vi "Write Plugin Connection Map.vi"(8 "error in (no error)":errorcluster, 10 "Plugin Connection Map":T1, 11 "CIF_UI in":refnum<class "CIF_UI.lvclass">) -> (0 "error out":errorcluster, 3 "CIF_UI out":refnum<class "CIF_UI.lvclass">)   [LabVIEW 2021, in "CIF_UI.lvclass"]
uses:
  CIF_UI.lvclass
  Typedef/Plugin Connection Map.ctl
  Typedef/Plugin Connections.ctl
  <vilib>/gRPC/LabVIEW gRPC Library/Shared/grpcId.ctl
  CIFPluginManager/CIFPluginManager/gRPC/CIF_Manager_client/RPC Messages/cif_manager_PluginInfo.ctl
  CIFPluginManager/CIFPluginManager/gRPC/CIF_Manager_client/RPC Messages/cif_manager_PluginVersion.ctl
  CIFPluginManager/CIFPluginManager/gRPC/CIF_Manager_client/RPC Messages/cif_plugincore_StatusData.ctl
  CIFPluginManager/CIFPluginManager/gRPC/CIF_Manager_client/RPC Messages/cif_plugincore_StatusData_State.ctl
  CIFPluginManager/CIFPluginManager/gRPC/CIF_Manager_client/RPC Messages/cif_plugincore_TimingStatistics.ctl
  CIFPluginManager/CIFPluginManager/gRPC/CIF_Manager_client/RPC Messages/cif_plugincore_TimingStatsBasic.ctl
  CIFPluginManager/CIFPluginManager/gRPC/CIF_Manager_client/RPC Messages/cif_plugincore_FifoStatistics.ctl
  CIFPluginManager/CIFPluginManager/gRPC/CIF_Manager_client/RPC Messages/cif_plugincore_Error.ctl
  CIFPluginManager/CIFPluginManager/gRPC/CIF_Manager_client/RPC Messages/cif_plugincore_MonitorDoubles.ctl
  CIFPluginManager/CIFPluginManager/gRPC/CIF_Manager_client/RPC Messages/cif_plugincore_MonitorU64.ctl
  CIFPluginManager/CIFPluginManager/gRPC/CIF_Manager_client/RPC Messages/cif_plugincore_MonitorI64.ctl
  CIF_UI.lvclass/CIF_UI.ctl
  CIFPluginManager/CIFPluginManager/gRPC/CIF_Manager_client/CIF_Manager_client.lvlib
  <vilib>/gRPC/LabVIEW gRPC Library/grpc-lvsupport-release.lvlib
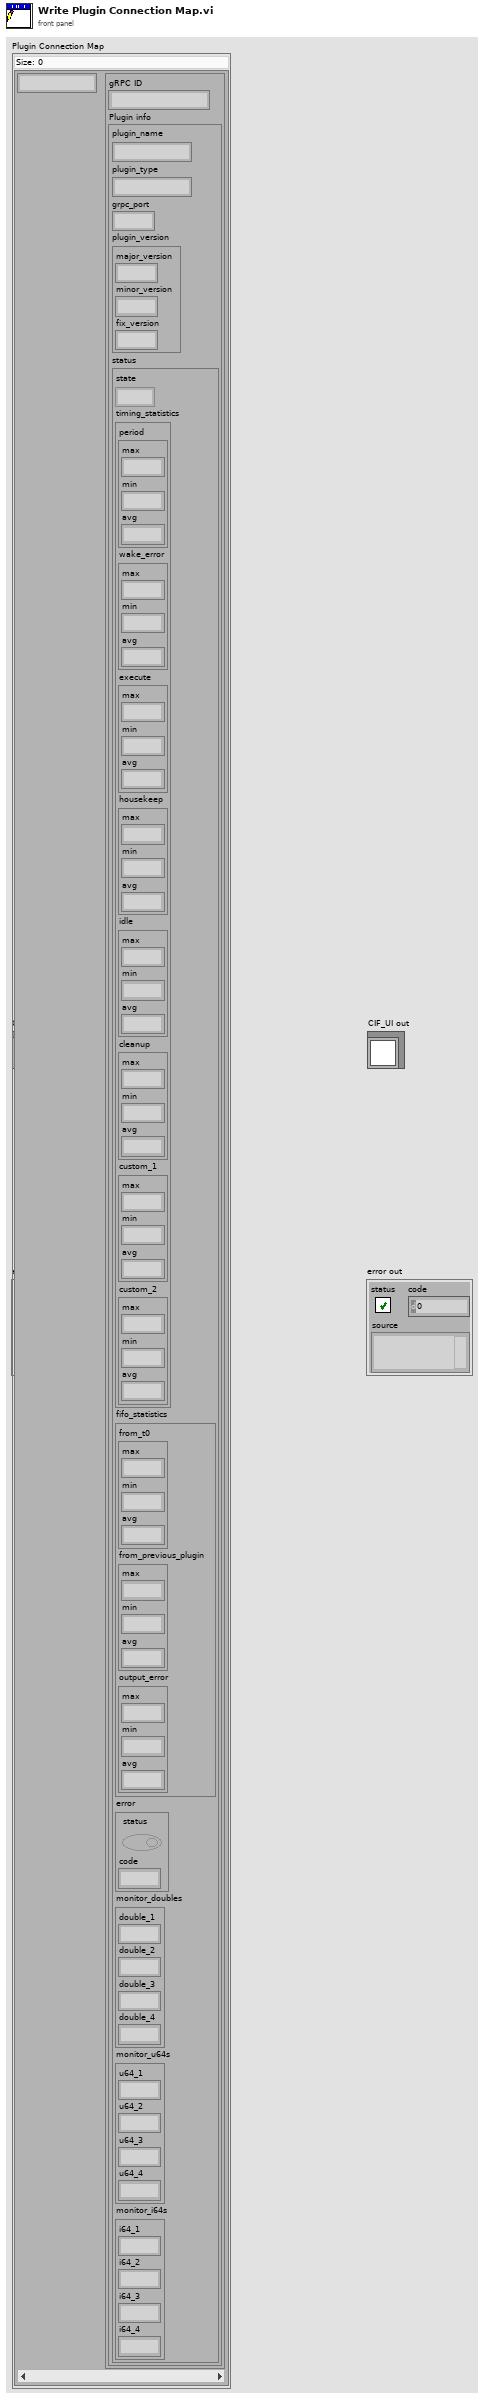
[diagram p1: front panel]
types:
  T1 = typedef "CIF_UI.lvclass/Plugin Connection Map.ctl" = map{string, T2}
  T2 = typedef "CIF_UI.lvclass/Plugin Connections.ctl" = cluster{"gRPC ID":T3, "Plugin info":T4}
  T3 = typedef "grpc-lvsupport-release.lvlib/grpcId.ctl" = u64
  T4 = typedef "CIF_Manager_client.lvlib/cif_manager_PluginInfo.ctl" = cluster{"plugin_name":string, "plugin_type":string, "grpc_port":i32, "plugin_version":T5, "status":T6}
  T5 = typedef "CIF_Manager_client.lvlib/cif_manager_PluginVersion.ctl" = cluster{"major_version":i32, "minor_version":i32, "fix_version":i32}
  T6 = typedef "CIF_Manager_client.lvlib/cif_plugincore_StatusData.ctl" = cluster{"state":T7, "timing_statistics":T8, "fifo_statistics":T10, "error":T11, "monitor_doubles":T12, "monitor_u64s":T13, "monitor_i64s":T14}
  T7 = typedef "CIF_Manager_client.lvlib/cif_plugincore_StatusData_State.ctl" = enum32{"NULL", "CREATING", "LISTENING", "RUNNING", "CLEANINGUP", "DESTROYING"}
  T8 = typedef "CIF_Manager_client.lvlib/cif_plugincore_TimingStatistics.ctl" = cluster{"period":T9, "wake_error":T9, "execute":T9, "housekeep":T9, "idle":T9, "cleanup":T9, "custom_1":T9, "custom_2":T9}
  T9 = typedef "CIF_Manager_client.lvlib/cif_plugincore_TimingStatsBasic.ctl" = cluster{"max":i64, "min":i64, "avg":dbl}
  T10 = typedef "CIF_Manager_client.lvlib/cif_plugincore_FifoStatistics.ctl" = cluster{"from_t0":T9, "from_previous_plugin":T9, "output_error":T9}
  T11 = typedef "CIF_Manager_client.lvlib/cif_plugincore_Error.ctl" = cluster{"status":bool, "code":i32}
  T12 = typedef "CIF_Manager_client.lvlib/cif_plugincore_MonitorDoubles.ctl" = cluster{"double_1":dbl, "double_2":dbl, "double_3":dbl, "double_4":dbl}
  T13 = typedef "CIF_Manager_client.lvlib/cif_plugincore_MonitorU64.ctl" = cluster{"u64_1":u64, "u64_2":u64, "u64_3":u64, "u64_4":u64}
  T14 = typedef "CIF_Manager_client.lvlib/cif_plugincore_MonitorI64.ctl" = cluster{"i64_1":i64, "i64_2":i64, "i64_3":i64, "i64_4":i64}
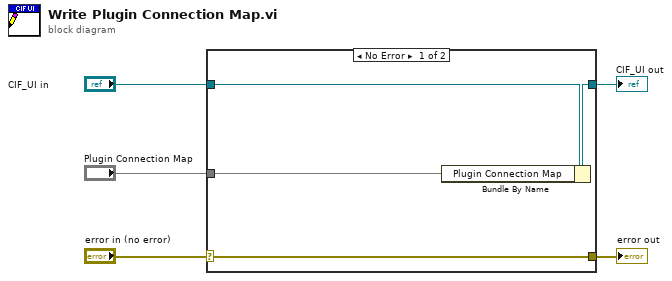
[diagram p0: block diagram]
diagram:
  n1 = case shown="No Error" "error in (no error)" {
    selector: "error in (no error)" -> [w9 w10]
    tunnel: [w9 w10] -> w4
    tunnel: [w7 w11] -> w2
    tunnel: "CIF_UI in" -> [w8 w11]
    tunnel: "Plugin Connection Map" -> [w6 _]
    frame No Error {
      n2 = Bundle By Name(cluster=w8, "Plugin Connection Map"=w6) -> (w7:refnum<class "CIF_UI.lvclass">)
    }
    frame Error {
    }
  }
  "error out" <- w4
  "CIF_UI out" <- w2
